vi "change2d.vi"(7 "reset(default false)":bool, 8 "index (col)":i32, 9 "index (row)":i32, 10 "read/write(T/F)":bool, 11 "2D Array":dbl[][](array[numeric])) -> (0 "result count":dbl, 3 "2D Array Result":dbl[][](array[numeric]))   [LabVIEW 2014]
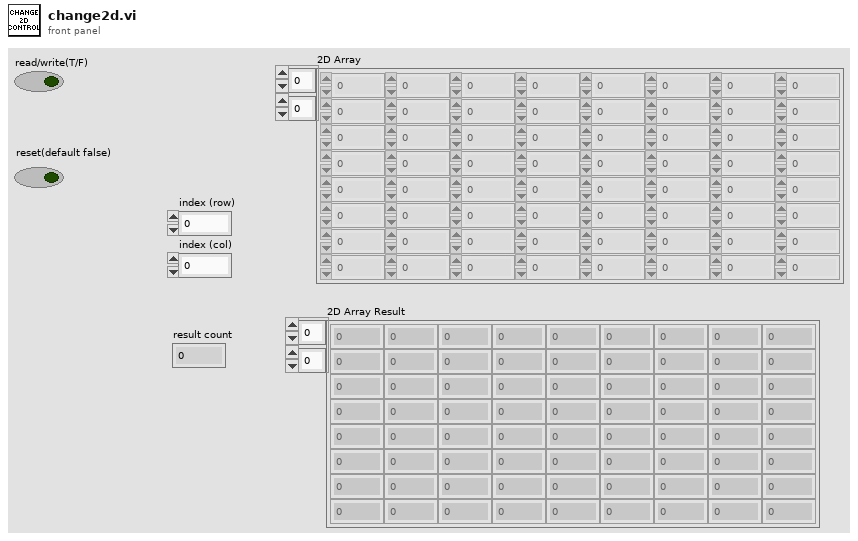
[diagram p1: front panel]
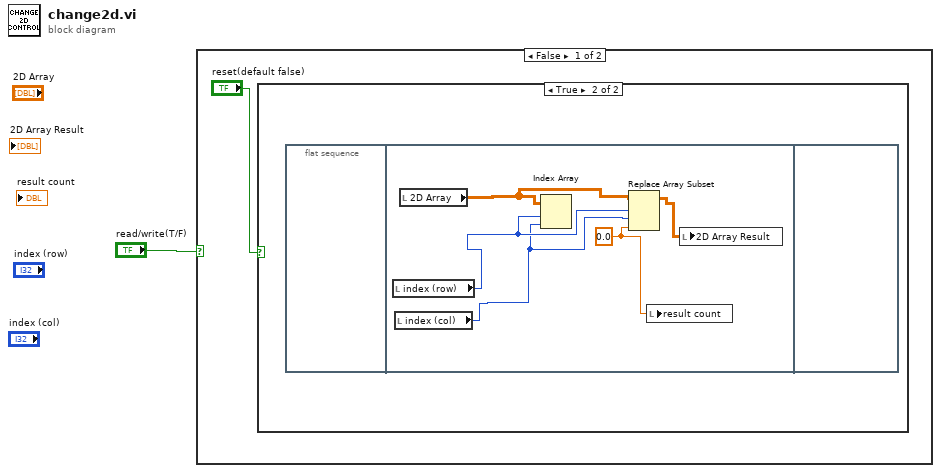
[diagram p0: block diagram]
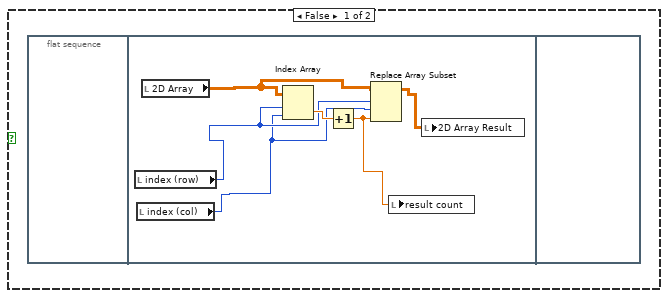
[diagram p2: hidden frame]
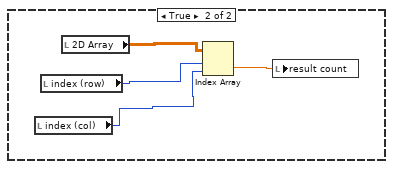
[diagram p3: hidden frame]
diagram:
  n1 = case shown="False" "read/write(T/F)" {
    frame False {
      n2 = case shown="True" "reset(default false)" {
        frame False {
          n3 = flat-sequence {
            frame #0 {
            }
            frame #1 {
              n4 = local read "index (row)"() -> (w4:i32)
              n5 = local read "index (col)"() -> (w3:i32)
              n6 = local read "2D Array"() -> (w8:dbl[][])
              n7 = Index Array(array=w8, index (row)=w4, index (col)=w3) -> (element=w7:dbl)
              n8 = Increment(x=w7) -> (x+1=w5:dbl)
              n9 = Replace Array Subset(array=w8, new element=w5, index (row)=w4, index (col)=w3) -> (w6:dbl[][])
              n10 = local write "result count"(w5) -> ()
              n11 = local write "2D Array Result"(w6) -> ()
            }
            frame #2 {
            }
          }
        }
        frame True {
          n12 = flat-sequence {
            frame #0 {
            }
            frame #1 {
              w9 = 0.0 ("new element/subarray")
              n13 = local read "index (row)"() -> (w11:i32)
              n14 = local read "index (col)"() -> (w10:i32)
              n15 = local read "2D Array"() -> (w13:dbl[][])
              n16 = Index Array(array=w13, index (row)=w11, index (col)=w10) -> ()  [unwired: 1 out]
              n17 = Replace Array Subset(array=w13, new element=w9, index (row)=w11, index (col)=w10) -> (w12:dbl[][])
              n18 = local write "result count"(w9) -> ()
              n19 = local write "2D Array Result"(w12) -> ()
            }
            frame #2 {
            }
          }
        }
      }
    }
    frame True {
      n20 = local read "index (col)"() -> (w15:i32)
      n21 = local read "index (row)"() -> (w16:i32)
      n22 = local read "2D Array"() -> (w17:dbl[][])
      n23 = Index Array(array=w17, index (row)=w16, index (col)=w15) -> (element=w14:dbl)
      n24 = local write "result count"(w14) -> ()
    }
  }
